vi "ThorLabsStage_Device.vi"(7 "Device-specific in":variant, 8 "error in (no error)":errorcluster, 10 "Position in":dbl[](array[numeric]), 11 "Operation":T2(ring)) -> (0 "error out":errorcluster, 1 "Device properties":cluster{"Axes":string[], "Tolerance":dbl[][]}, 2 "Position out":dbl[](array[numeric]), 3 "Status":T1, 5 "Device-specific out":variant)   [LabVIEW 2018]
panel:
  in  "MG17Motor 3":refnum<k7>(container)
  in  "MG17Motor 2":refnum<k7>(container)
  in  "MG17Motor":refnum<k7>(container)
  in  "MG17System":refnum<k7>(container)
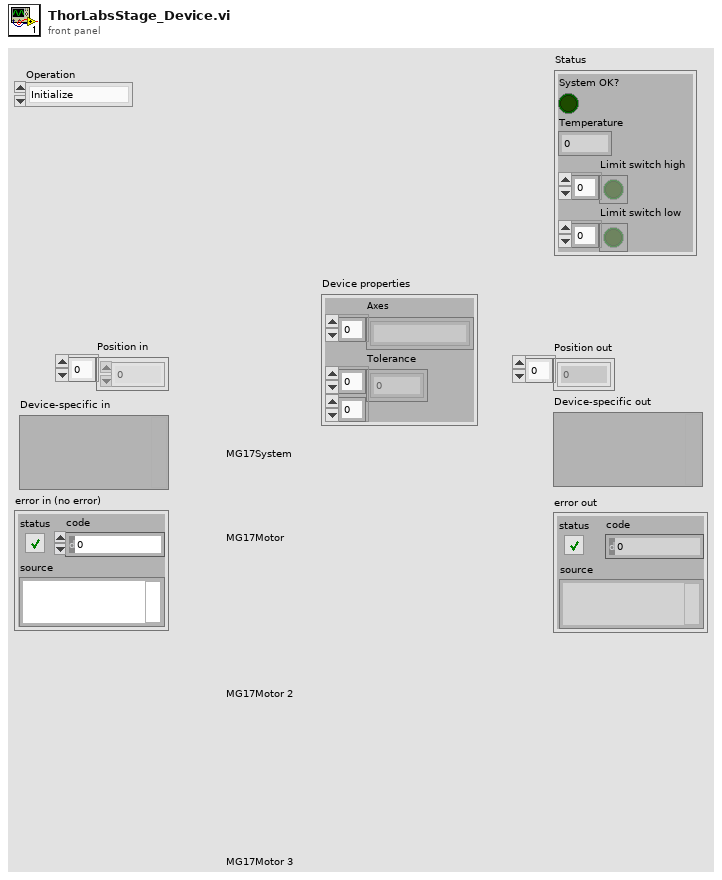
[diagram p1: front panel]
types:
  T1 = cluster{"System OK?":bool, "Temperature":dbl, "Limit switch high":bool[], "Limit switch low":bool[]}
  T2 = enum16{"Initialize", "Shut down", "Set position", "Get position", "Get status", "Other settings"}
  T3 = cluster{"Axis parameters":cluster{"IHWType":i32, "Serial number":i32, "MG17Motor":refnum<k7>}[], "Stage thresholds":cluster{string[], dbl[][]}}
  T4 = cluster{"IHWType":i32, "Serial number":i32, "MG17Motor":refnum<k7>}
  T5 = cluster{"IHWType":i32, "Serial number":i32, "MG17Motor":refnum<k7>}[]
  T6 = cluster{cluster{"IHWType":i32, "Serial number":i32, "MG17Motor":refnum<k7>}[], cluster{string[], dbl[][]}}
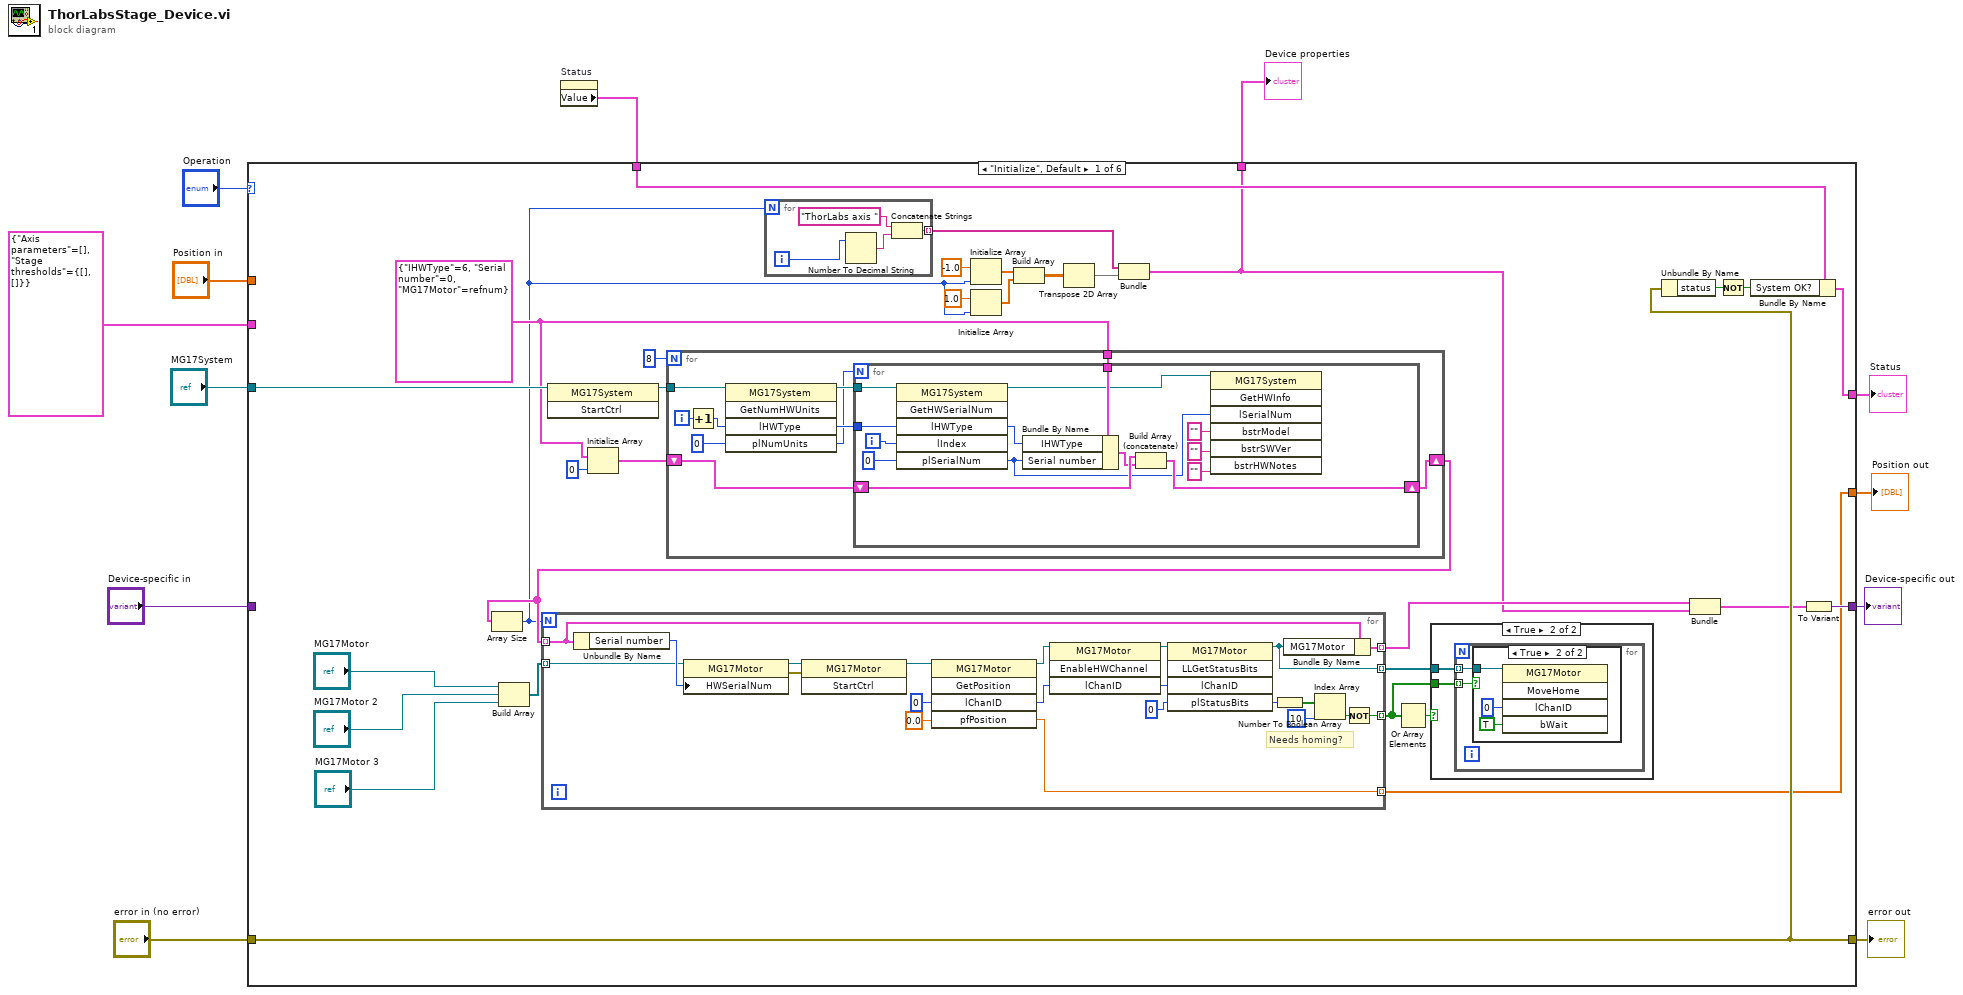
[diagram p0: block diagram]
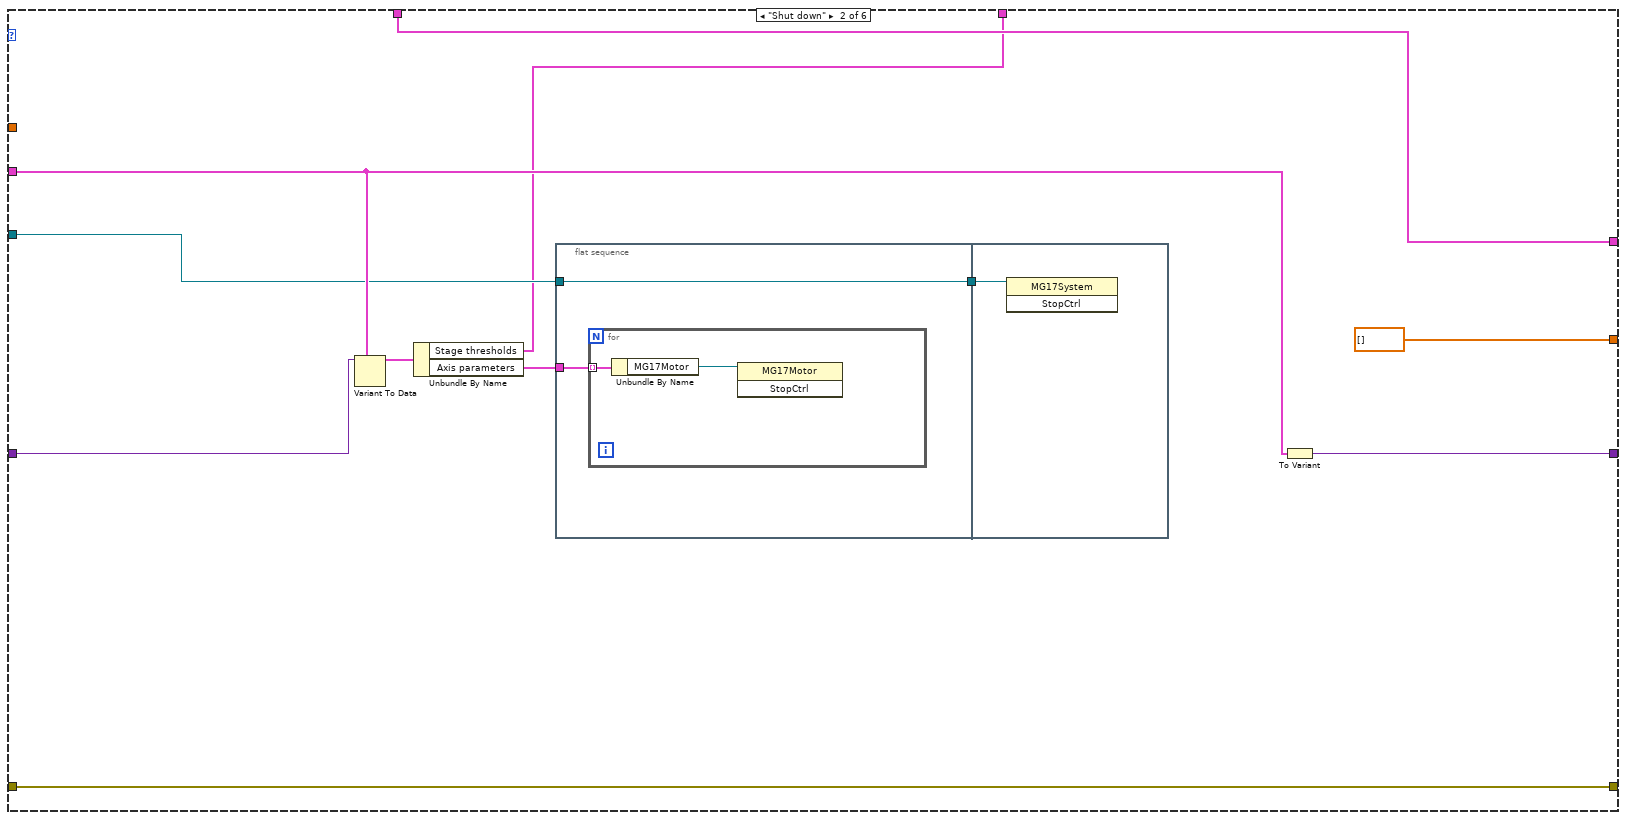
[diagram p4: hidden frame]
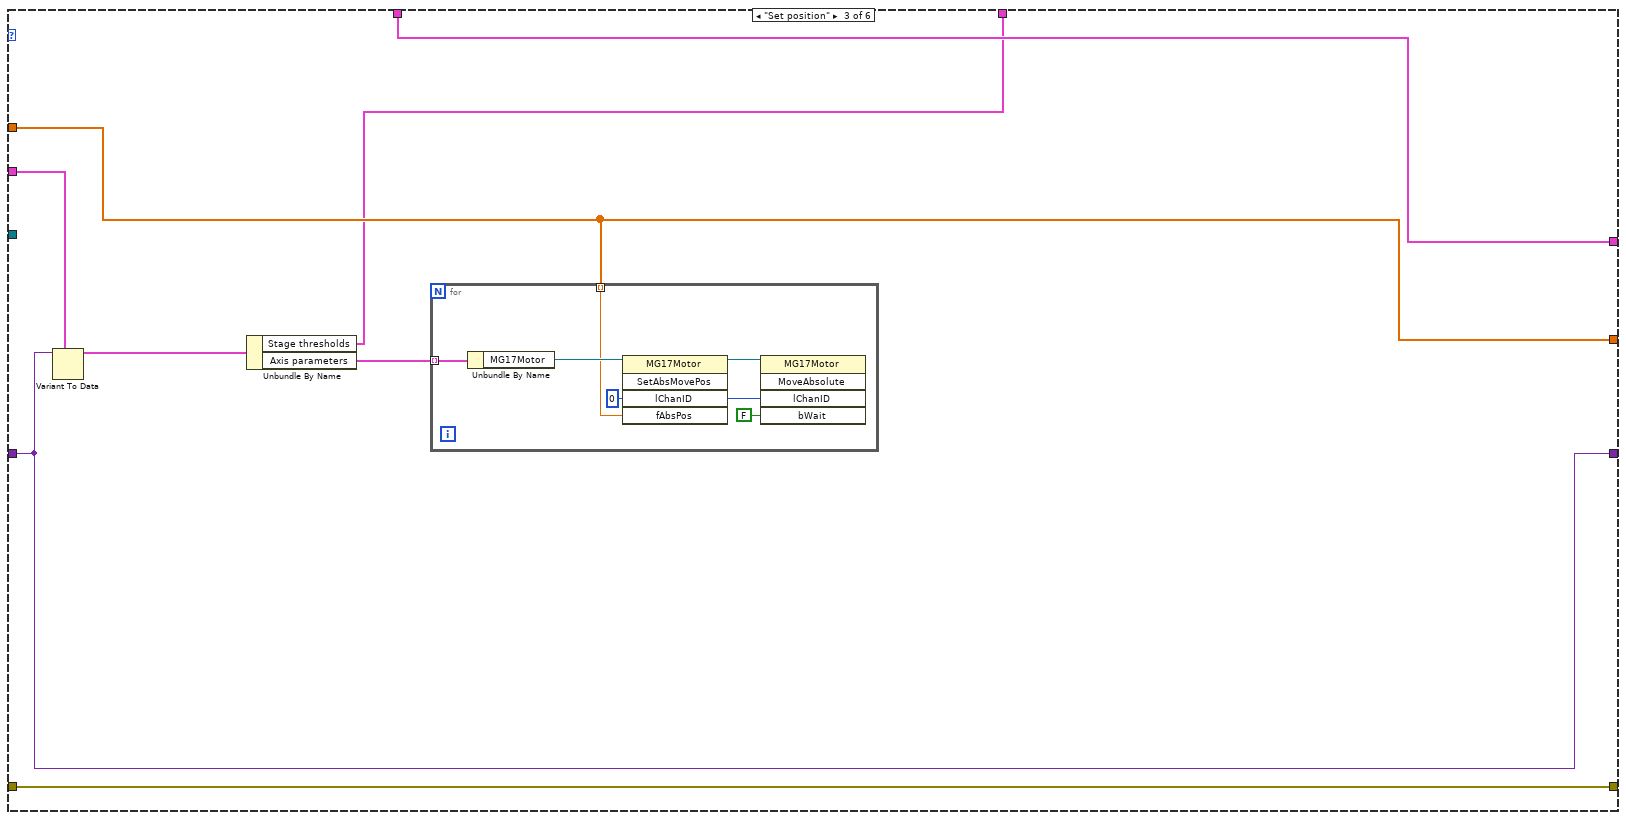
[diagram p5: hidden frame]
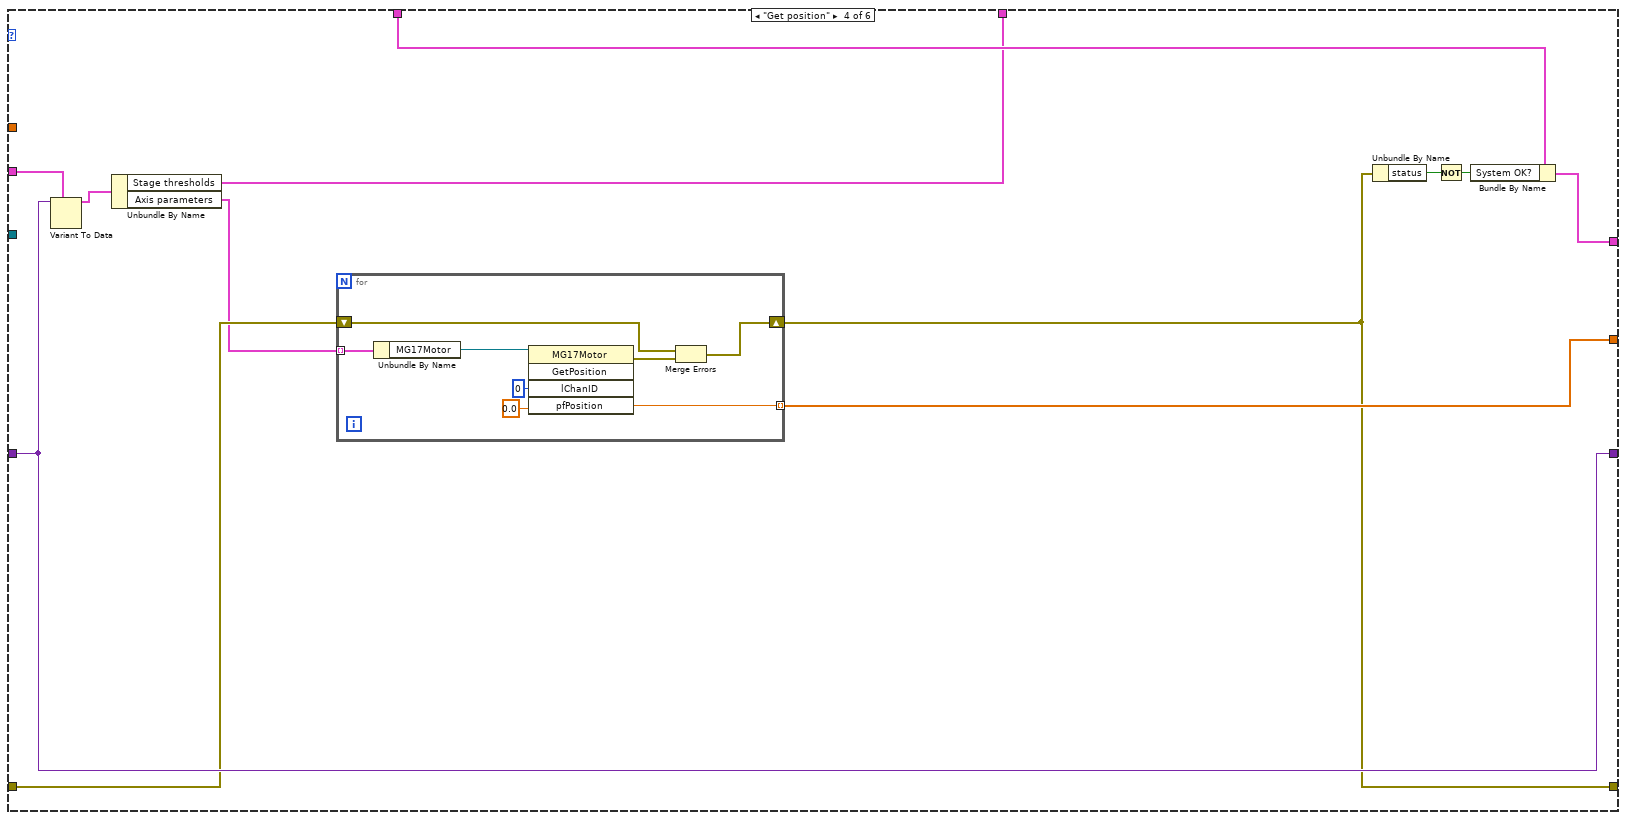
[diagram p6: hidden frame]
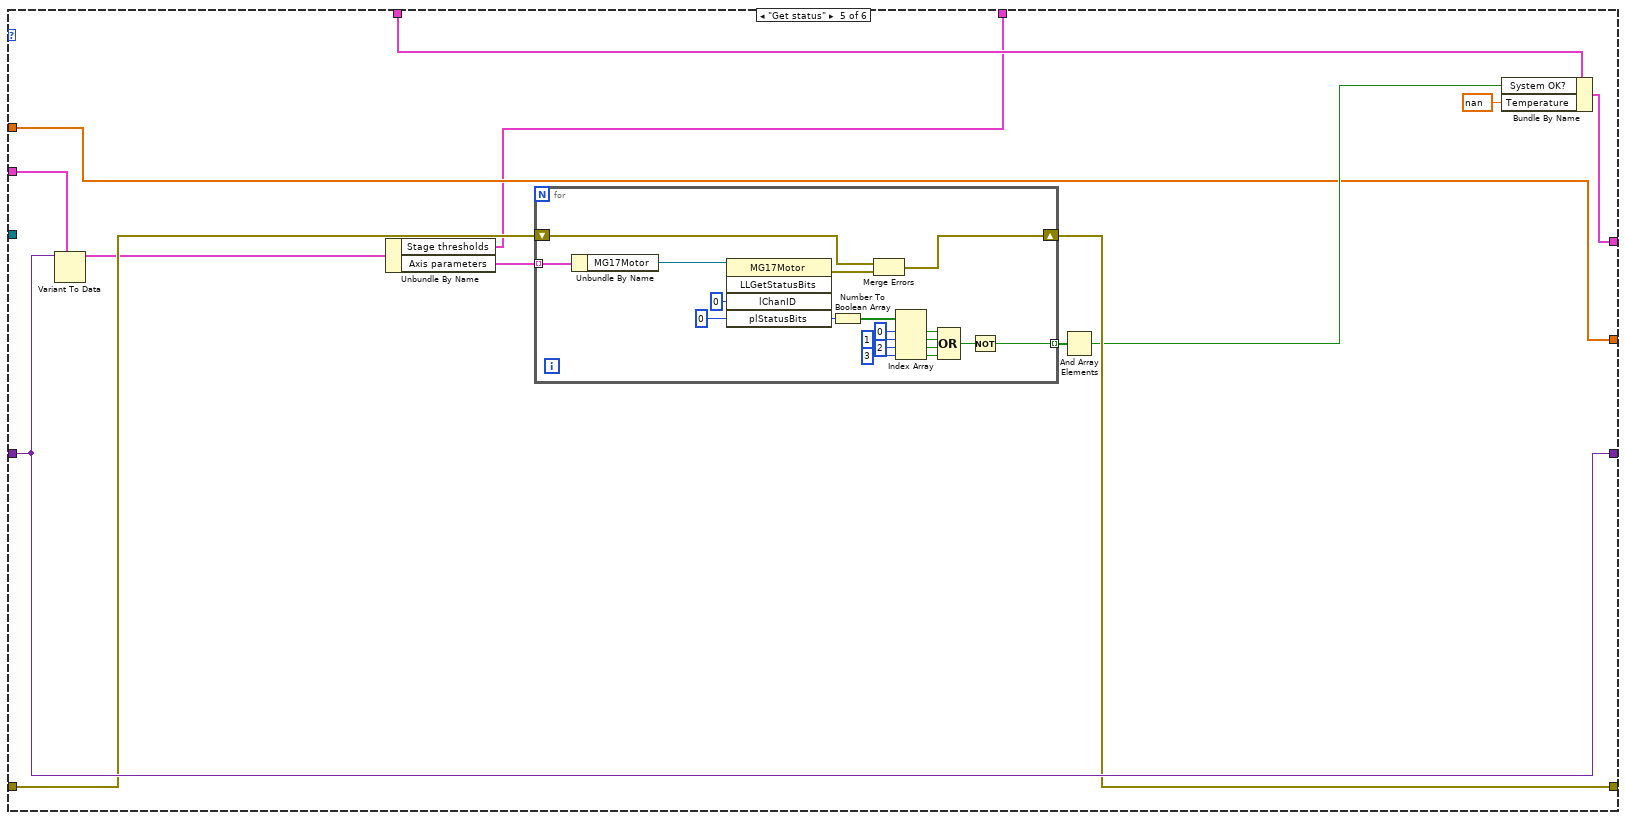
[diagram p7: hidden frame]
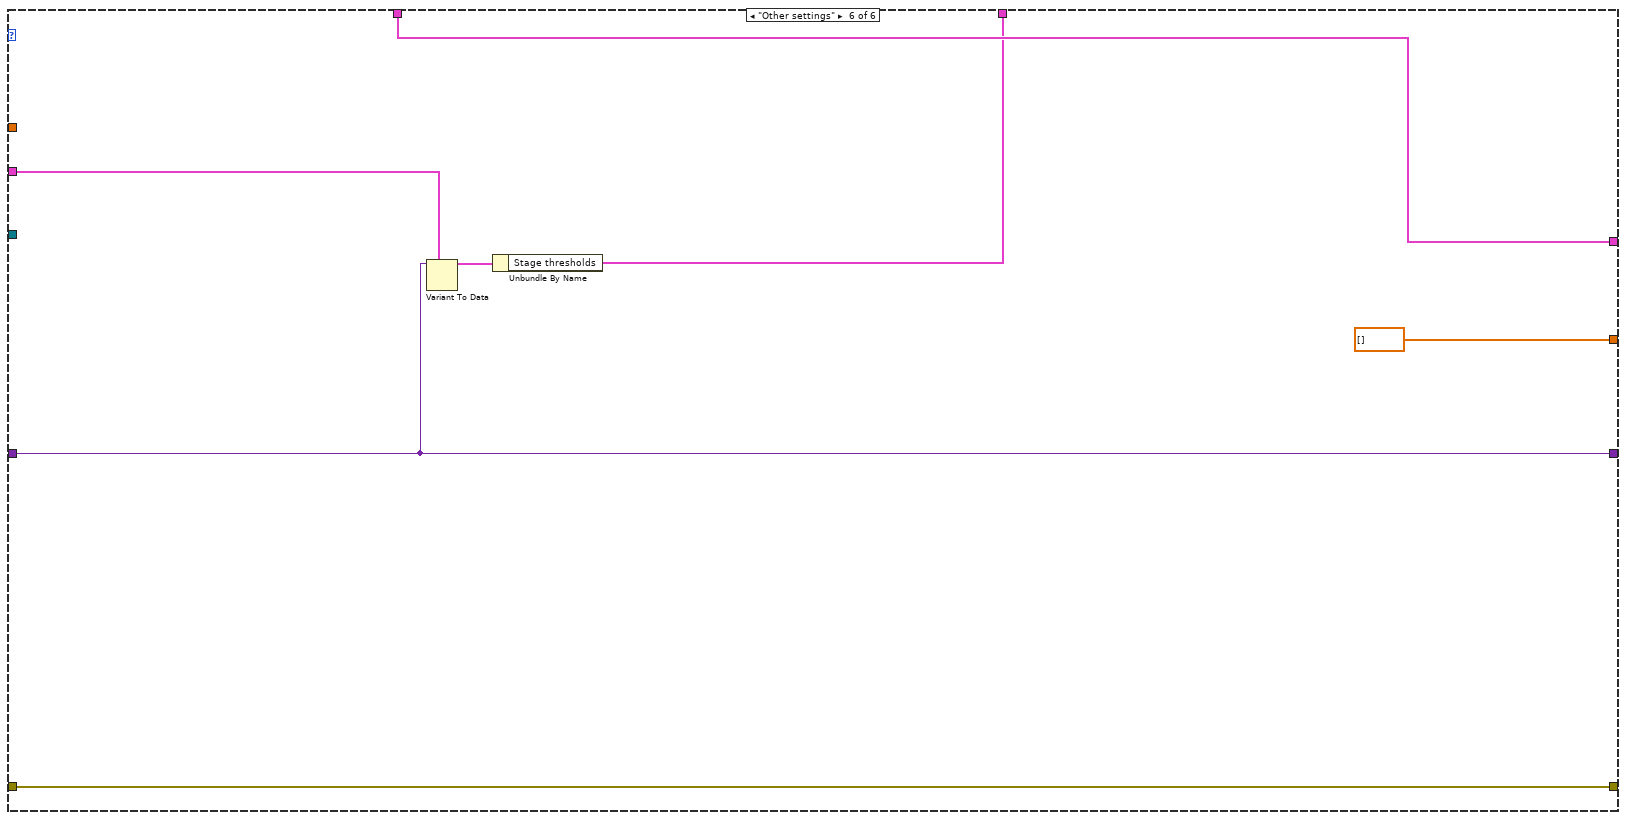
[diagram p8: hidden frame]
diagram:
  n1 = property on="Status" class="Clust (strict)"() -> ("Value"=w11:T1)  [unwired: 2 in, 2 out]
  n2 = case shown="\"Initialize\", Default" "Operation" {
    tunnel: "Position in" -> [_ _ w120 _ w155 _]
    tunnel: w11 -> [w44 w111 w124 w141 w164 w190]
    tunnel: [w43 w111 w124 w140 w163 w190] -> w10
    tunnel: "Device-specific in" -> [_ w108 w121 w143 w161 w187]
    tunnel: [w22 dbl[] [] ("Position in") w120 w137 w155 dbl[] [] ("Position in")] -> w7
    tunnel: [w42 w106 w121 w143 w161 w187] -> w6
    tunnel: [w30 w110 w123 w135 w158 w189] -> w5
    tunnel: "error in (no error)" -> [w30 w110 w123 w136 w159 w189]
    tunnel: T3 {"Axis parameters"=[], "Stage thresholds"={[], []}} -> [_ w107 w122 w142 w160 w186]
    tunnel: "MG17System" -> [w41 w104 _ _ _ _]
    tunnel: [w15 w101 w117 w133 w152 w184] -> w2
    frame "Initialize", Default {
      w36 = T4 {"IHWType"=6, "Serial number"=0, "MG17Motor"=refnum}
      n3 = Build Array("MG17Motor", "MG17Motor 2", "MG17Motor 3") -> (w27:refnum<k7>[])
      n4 = invoke class="MG17System" method="StartCtrl"(reference=w41) -> (reference out=w38:refnum<k7>)  [unwired: 2 in, 2 out]
      n5 = Initialize Array(w36, 0 ("dimension size")) -> (w34:T5)
      n6 = for {
        N: 8 -> [_]
        tunnel: w38 -> [w86]
        shift-right: [w77] -> w24
        shift-left: w34 -> [w78]
        tunnel: w36 -> [w79]
        i -> [w81]
        n7 = Increment(x=w81) -> (x+1=w80:i32)
        n8 = invoke class="MG17System" method="GetNumHWUnits"(reference=w86, "lHWType"=w80, "plNumUnits"=0) -> (reference out=w84:refnum<k7>, "lHWType"=w83:i32, "plNumUnits"=w82:i32)  [unwired: 2 in, 2 out]
        n9 = for {
          N: w82 -> [_]
          tunnel: w84 -> [w100]
          tunnel: w83 -> [w99]
          tunnel: w79 -> [w96]
          shift-right: [w93] -> w77
          shift-left: w78 -> [w94]
          i -> [w97]
          n10 = invoke class="MG17System" method="GetHWSerialNum"(reference=w100, "lHWType"=w99, "lIndex"=w97, "plSerialNum"=0) -> (reference out=w91:refnum<k7>, "lHWType"=w95:i32, "plSerialNum"=w90:i32)  [unwired: 2 in, 3 out]
          n11 = Bundle By Name(cluster=w96, "IHWType"=w95, "Serial number"=w90) -> (w92:T4)
          n12 = Build Array (concatenate)(w94, w92) -> (w93:T5)
          n13 = invoke class="MG17System" method="GetHWInfo"(reference=w91, "lSerialNum"=w90, "bstrModel"="", "bstrSWVer"="", "bstrHWNotes"="") -> ()  [unwired: 2 in, 7 out]
        }
      }
      n14 = Array Size(array=w24) -> (size(s)=w19:i32)
      n15 = for {
        N: w19 -> [_]
        tunnel: w24 -> [w69] mode=indexing
        tunnel: w27 -> [w70] mode=indexing
        tunnel: [w63] -> w22 mode=indexing
        tunnel: [w68] -> w16 mode=indexing
        tunnel: [w56] -> w25 mode=indexing
        tunnel: [w57] -> w23 mode=indexing
        # "Needs homing?"
        n16 = Unbundle By Name(w69) -> ("Serial number"=w76:i32)
        n17 = property class="MG17Motor"(reference=w70, "HWSerialNum"=w76) -> (reference out=w75:refnum<k7>, error out=w74:errorcluster)  [unwired: 1 in]
        n18 = invoke class="MG17Motor" method="StartCtrl"(reference=w75, error in=w74) -> (reference out=w73:refnum<k7>)  [unwired: 1 in, 2 out]
        n19 = invoke class="MG17Motor" method="GetPosition"(reference=w73, "lChanID"=0, "pfPosition"=sgl 0.0) -> (reference out=w67:refnum<k7>, "lChanID"=w66:i32, "pfPosition"=w63:sgl)  [unwired: 2 in, 2 out]
        n20 = invoke class="MG17Motor" method="EnableHWChannel"(reference=w67, "lChanID"=w66) -> (reference out=w65:refnum<k7>, "lChanID"=w64:i32)  [unwired: 2 in, 2 out]
        n21 = invoke class="MG17Motor" method="LLGetStatusBits"(reference=w65, "lChanID"=w64, "plStatusBits"=0) -> (reference out=w57:refnum<k7>, "plStatusBits"=w61:i32)  [unwired: 2 in, 3 out]
        n22 = Number To Boolean Array(number=w61) -> (Boolean array=w60:bool[])
        n23 = Bundle By Name(cluster=w69, "MG17Motor"=w57) -> (w68:T4)
        n24 = Index Array(array=w60, index=10) -> (element=w58:bool)
        n25 = Not(x=w58) -> (.not. x?=w56:bool)
      }
      n26 = for {
        N: w19 -> [_]
        tunnel: [w45] -> w18 mode=indexing
        i -> [w48]
        n27 = Number To Decimal String(number=w48) -> (decimal integer string=w47:string)  [unwired: 1 in]
        n28 = Concatenate Strings("ThorLabs axis ", w47) -> (w45:string)
      }
      n29 = Initialize Array(-1.0 ("element"), w19) -> (w29:dbl[])
      n30 = Initialize Array(1.0 ("element"), w19) -> (w20:dbl[])
      n31 = Build Array(w29, w20) -> (w17:dbl[][])
      n32 = Transpose 2D Array(2D array=w17) -> (transposed array=w13:dbl[][])
      n33 = Bundle(w18, w13) -> (w15:cluster{string[], dbl[][]})  [unwired: 1 in]
      n34 = Or Array Elements(Boolean array=w25) -> (logical OR=w26:bool)
      n35 = case shown="True" w26 {
        tunnel: w25 -> [_ w49]
        tunnel: w23 -> [_ w50]
        frame False {
        }
        frame True {
          n36 = for {
            tunnel: w50 -> [w51] mode=indexing
            tunnel: w49 -> [w52] mode=indexing
            n37 = case shown="True" w52 {
              tunnel: w51 -> [_ w54]
              frame False {
              }
              frame True {
                n38 = invoke class="MG17Motor" method="MoveHome"(reference=w54, "lChanID"=0, "bWait"=TRUE) -> ()  [unwired: 2 in, 5 out]
              }
            }
          }
        }
      }
      n39 = Unbundle By Name(w30) -> ("status"=w40:bool)
      n40 = Bundle(w16, w15) -> (w14:T6)  [unwired: 1 in]
      n41 = Not(x=w40) -> (.not. x?=w39:bool)
      n42 = Bundle By Name(cluster=w44, "System OK?"=w39) -> (w43:T1)
      n43 = To Variant(anything=w14) -> (Variant=w42:variant)
    }
    frame "Shut down" {
      n44 = Variant To Data(type=w107, Variant=w108) -> (data=w103:T3)  [unwired: 1 in, 1 out]
      n45 = Unbundle By Name(w103) -> ("Stage thresholds"=w101:cluster{string[], dbl[][]}, "Axis parameters"=w102:T5)
      n46 = flat-sequence {
        tunnel: w102 -> [w113]
        tunnel: [w112] -> w105
        tunnel: w104 -> [w112]
        tunnel: w105 -> [w116]
        frame #0 {
          n47 = for {
            tunnel: w113 -> [w115] mode=indexing
            n48 = Unbundle By Name(w115) -> ("MG17Motor"=w114:refnum<k7>)
            n49 = invoke class="MG17Motor" method="StopCtrl"(reference=w114) -> ()  [unwired: 2 in, 3 out]
          }
        }
        frame #1 {
          n50 = invoke class="MG17System" method="StopCtrl"(reference=w116) -> ()  [unwired: 2 in, 3 out]
        }
      }
      n51 = To Variant(anything=w107) -> (Variant=w106:variant)
    }
    frame "Set position" {
      n52 = Variant To Data(type=w122, Variant=w121) -> (data=w119:T3)  [unwired: 1 in, 1 out]
      n53 = Unbundle By Name(w119) -> ("Stage thresholds"=w117:cluster{string[], dbl[][]}, "Axis parameters"=w118:T5)
      n54 = for {
        tunnel: w118 -> [w131] mode=indexing
        tunnel: w120 -> [w125] mode=indexing
        n55 = Unbundle By Name(w131) -> ("MG17Motor"=w129:refnum<k7>)
        n56 = invoke class="MG17Motor" method="SetAbsMovePos"(reference=w129, "lChanID"=0, "fAbsPos"=w125) -> (reference out=w128:refnum<k7>, "lChanID"=w126:i32)  [unwired: 2 in, 3 out]
        n57 = invoke class="MG17Motor" method="MoveAbsolute"(reference=w128, "lChanID"=w126, "bWait"=FALSE) -> ()  [unwired: 2 in, 5 out]
      }
    }
    frame "Get position" {
      n58 = Variant To Data(type=w142, Variant=w143) -> (data=w134:T3)  [unwired: 1 in, 1 out]
      n59 = Unbundle By Name(w134) -> ("Stage thresholds"=w133:cluster{string[], dbl[][]}, "Axis parameters"=w132:T5)
      n60 = for {
        tunnel: w132 -> [w151] mode=indexing
        tunnel: [w148] -> w137 mode=indexing
        shift-right: [w146] -> w135
        shift-left: w136 -> [w145]
        n61 = Unbundle By Name(w151) -> ("MG17Motor"=w150:refnum<k7>)
        n62 = invoke class="MG17Motor" method="GetPosition"(reference=w150, "lChanID"=0, "pfPosition"=sgl 0.0) -> (error out=w147:errorcluster, "pfPosition"=w148:sgl)  [unwired: 2 in, 3 out]
        n63 = Merge Errors(w145, w147) -> (w146:errorcluster)
      }
      n64 = Unbundle By Name(w135) -> ("status"=w139:bool)
      n65 = Not(x=w139) -> (.not. x?=w138:bool)
      n66 = Bundle By Name(cluster=w141, "System OK?"=w138) -> (w140:T1)
    }
    frame "Get status" {
      n67 = Variant To Data(type=w160, Variant=w161) -> (data=w154:T3)  [unwired: 1 in, 1 out]
      n68 = Unbundle By Name(w154) -> ("Stage thresholds"=w152:cluster{string[], dbl[][]}, "Axis parameters"=w153:T5)
      n69 = for {
        tunnel: w153 -> [w183] mode=indexing
        shift-right: [w179] -> w158
        shift-left: w159 -> [w178]
        tunnel: [w165] -> w157 mode=indexing
        n70 = Unbundle By Name(w183) -> ("MG17Motor"=w182:refnum<k7>)
        n71 = invoke class="MG17Motor" method="LLGetStatusBits"(reference=w182, "lChanID"=0, "plStatusBits"=0) -> (error out=w180:errorcluster, "plStatusBits"=w176:i32)  [unwired: 2 in, 3 out]
        n72 = Number To Boolean Array(number=w176) -> (Boolean array=w175:bool[])
        n73 = Merge Errors(w178, w180) -> (w179:errorcluster)
        n74 = Index Array(array=w175, index #1=0 ("index"), index #2=1 ("index"), index #3=2 ("index"), index #4=3 ("index")) -> (element #1=w170:bool, element #2=w169:bool, element #3=w168:bool, element #4=w167:bool)
        n75 = Compound Arithmetic op=OR(w170, w169, w168, w167) -> (w166:bool)
        n76 = Not(x=w166) -> (.not. x?=w165:bool)
      }
      n77 = And Array Elements(Boolean array=w157) -> (logical AND=w156:bool)
      n78 = Bundle By Name(cluster=w164, "System OK?"=w156, "Temperature"=nan) -> (w163:T1)
    }
    frame "Other settings" {
      n79 = Variant To Data(type=w186, Variant=w187) -> (data=w185:T3)  [unwired: 1 in, 1 out]
      n80 = Unbundle By Name(w185) -> ("Stage thresholds"=w184:cluster{string[], dbl[][]})
    }
  }
  "Status" <- w10
  "Device-specific out" <- w6
  "error out" <- w5
  "Position out" <- w7
  "Device properties" <- w2
